vi "AddFunction (SubVI).vi"(8 "comm?":bool, 9 "RangeChB":T1(ring) caption="Диапазон \"B\"", 10 "RangeChA":T2(ring) caption="Диапазон \"A\"", 11 "Table in":refnum<vi>) -> ()   [LabVIEW 2017]
uses:
  st_str Global.vi
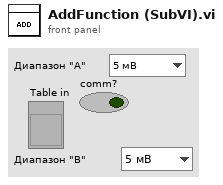
[diagram p1: front panel]
types:
  T1 = enum16{"5 мВ", "10 мВ", "25 мВ", "50 мВ", "100 мВ", "250 мВ", "0,5 В", "1 В", "2,5 В", "5 В", "10 В", "Авто", "Выкл."}
  T2 = enum16{"5 мВ", "10 мВ", "25 мВ", "50 мВ", "100 мВ", "250 мВ", "0,5 В", "1,0 В", "2,5 В", "5 В", "10 В", "Авто", "Выкл."}
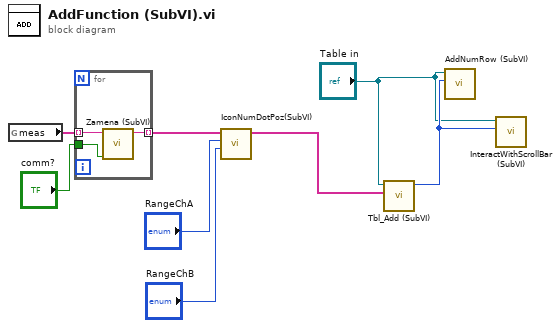
[diagram p0: block diagram]
diagram:
  n1 = global read "st_str Global.vi" "meas"() -> (w3:string[])
  n2 = for {
    tunnel: w3 -> [w11] mode=indexing
    tunnel: [w10] -> w2 mode=indexing
    tunnel: "comm?" -> [w9]
    n3 = call "Zamena (SubVI).vi"("comm?"=w9, "input string"=w11) -> ("result string 2"=w10:string)  [unwired: 9 in]
  }
  n4 = call "IconNumDotPoz(SubVI).vi"("RangeChB"="RangeChB", "RangeChA"="RangeChA", "meas"=w2) -> ("meas 2"=w6:string[])  [unwired: 8 in]
  n5 = call "Tbl_Add (SubVI).vi"("meas"=w6, "Table in"="Table in") -> ("element"=w8:i32)  [unwired: 9 in]
  n6 = call "AddNumRow (SubVI).vi"("element"=w8, "Table in"="Table in") -> ()  [unwired: 10 in]
  n7 = call "InteractWithScrollBar (SubVI).vi"("element"=w8, "Table in"="Table in") -> ()  [unwired: 10 in]
